vi "Supply_ReadCurrent.vi"(8 "error in (no error)":errorcluster, 11 "KE236 in":refnum<class "KE236.lvclass">) -> (0 "error out":errorcluster, 2 "Current in nA":dbl format="%#.6g", 3 "KE236 out":refnum<class "KE236.lvclass">)   [LabVIEW 2018, in "KE236.lvclass"]
uses:
  KE236.lvclass
  <vilib>/regexp/Match Regular Expression.xnode
  InstrControl.lvclass
panel:
  out "compliance letter":string
  out "Status string":string
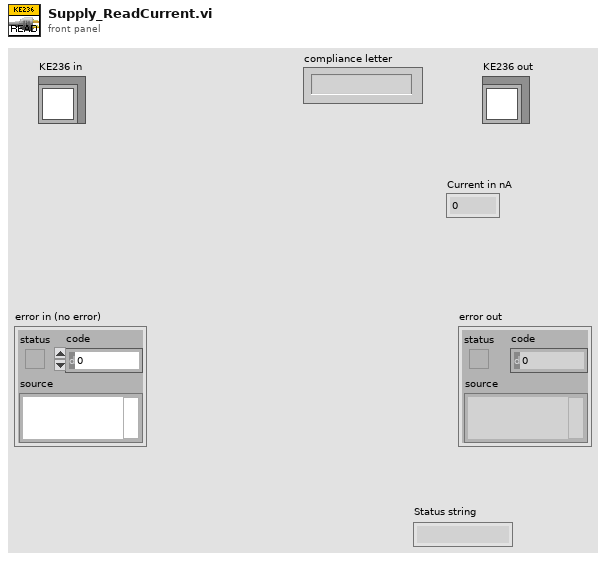
[diagram p1: front panel]
types:
  T1 = cluster{"error":bool, "code":i32, "source":string}
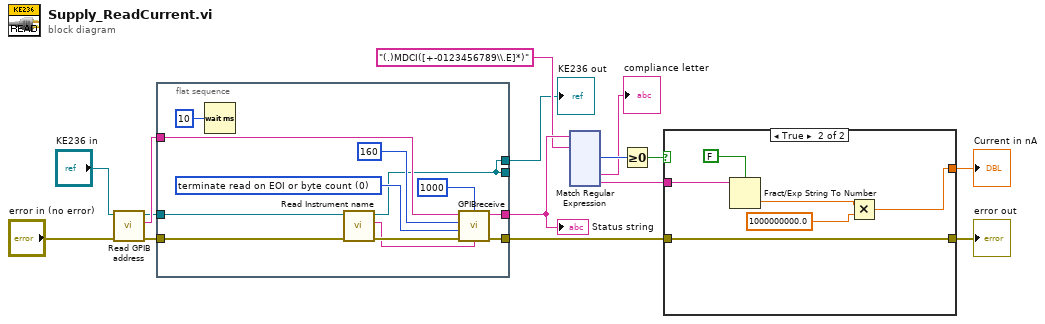
[diagram p0: block diagram]
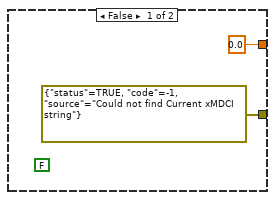
[diagram p2: hidden frame]
diagram:
  n1 = call-dynamic "Read GPIB address.vi"("error in (no error)"="error in (no error)", "InstControl in"="KE236 in") -> ("error out"=w11:errorcluster, "GPIB address"=w12:string, "InstControl out"=w10:refnum<class "KE236.lvclass">)  [unwired: 7 in]
  n2 = flat-sequence {
    tunnel: w12 -> [w27]
    tunnel: w11 -> [w19]
    tunnel: [w22] -> w15
    tunnel: [w21] -> w8
    tunnel: w10 -> [w20]
    tunnel: [w16] -> _
    tunnel: [w16] -> w1
    frame #0 {
      w24 = 0 items=["terminate read on EOI or byte count", "terminate read on EOI, byte count, or CR", "terminate read on EOI, byte count, or LF"] ("read mode")
      n3 = Wait (ms)(milliseconds to wait=u32 10) -> ()  [unwired: 1 out]
      n4 = call-dynamic "Read Instrument name.vi"("error in (no error)"=w19, "InstControl in"=w20) -> ("error out"=w18:errorcluster, "Instrument name"=w17:string, "InstControl out"=w16:refnum<class "KE236.lvclass">)  [unwired: 7 in]
      n5 = call "GPIBreceive.vi"("timeout ms"=u32 1000, "address string"=w27, "byte count"=160, "source"=w17, "read mode"=w24, "error in"=w18) -> ("read buffer"=w22:string, "error out"=w21:T1)  [unwired: 1 in, 1 out]
    }
  }
  n6 = xnode "Match Regular Expression"("input string"=w15, "regular expression"="(.)MDCI([+-0123456789\\.E]*)") -> ("offset past match"=w13:i32, "submatch 1"=→"compliance letter":string, "submatch 2"=w4:string)  [unwired: 4 in, 4 out]
  n7 = Greater Or Equal To 0?(x=w13) -> (x >= 0?=w14:bool)
  n8 = case shown="True" w14 {
    tunnel: [errorcluster {"status"=TRUE, "code"=-1, "source"="Could not find Current xMDCI string"} ("error out") w33] -> w5
    tunnel: w8 -> [_ w33]
    tunnel: w4 -> [_ w35]
    tunnel: [0.0 w30] -> w2
    frame False {
      (unwired) FALSE ("Compliance exceeded?")
    }
    frame True {
      n9 = Fract/Exp String To Number(use system decimal point (T)=FALSE, string=w35) -> (number=w32:dbl)  [unwired: 2 in, 1 out]
      n10 = Multiply(x=w32, y=1000000000.0 ("number")) -> (x*y=w30:dbl)
    }
  }
  "error out" <- w5
  "Current in nA" <- w2
  "KE236 out" <- w1
  "Status string" <- w15
